vi "Test Criteria, Format Comments.vi"(8 "error in":errorcluster, 11 "Tbl Refnum":refnum<vi>) -> (0 "error out":errorcluster, 3 "Tbl Refnum out":refnum<vi>)   [LabVIEW 2010]
uses:
  <vilib>/Utility/miscctls.llb/LVRowAndColumnTypeDef.ctl
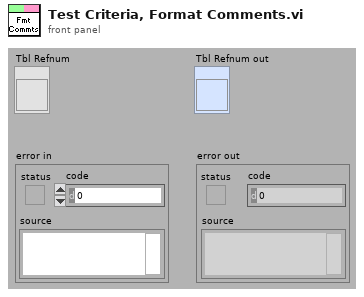
[diagram p1: front panel]
types:
  T1 = typedef "LVRowAndColumnTypeDef.ctl" = cluster{"Row":i32, "Column":i32}
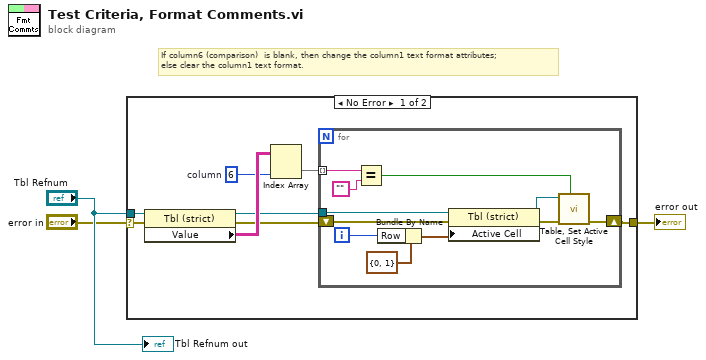
[diagram p0: block diagram]
diagram:
  # "If column6 (comparison)  is blank, then change the column1 text format attributes;\nelse clear the column1 text format."
  n1 = case shown="No Error" "error in" {
    selector: "error in" -> [w4 w23]
    tunnel: "Tbl Refnum" -> [w9 _]
    tunnel: [w6 w23] -> w2
    frame No Error {
      w5 = 6  # column
      n2 = property class="Tbl (strict)"(reference=w9, error in=w4) -> (reference out=w7:refnum<vi>, error out=w8:errorcluster, "Value"=w11:string[][])
      n3 = Index Array(array=w11, index (col)=w5) -> (element=w10:string[])  [unwired: 1 in]
      n4 = for {
        tunnel: w10 -> [w22] mode=indexing
        shift-right: [w14] -> w6
        shift-left: w8 -> [w15]
        tunnel: w7 -> [w13]
        i -> [w19]
        n5 = Equal?(x=w22, y="") -> (x = y?=w12:bool)
        n6 = Bundle By Name(cluster=T1 {"Row"=0, "Column"=1} ("Selection Start 2"), "Row"=w19) -> (w18:T1)
        n7 = property class="Tbl (strict)"(reference=w13, error in=w15, "Active Cell"=w18) -> (reference out=w16:refnum<vi>, error out=w17:errorcluster)
        n8 = call "Table, Set Active Cell Style.vi"("Enable (T)"=w12, "error in"=w17, "Tbl Refnum"=w16) -> ("error out"=w14:errorcluster)  [unwired: 5 in, 1 out]
      }
    }
    frame Error {
    }
  }
  "error out" <- w2
  "Tbl Refnum out" <- "Tbl Refnum"
